vi "zero_FGV.vi"(7 "comandos":enum16{"Set", "Zerar?"}(ring)=enum."Zerar?", 11 "Value":bool) -> (3 "Zerar?":bool)   [LabVIEW 2018]
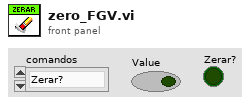
[diagram p1: front panel]
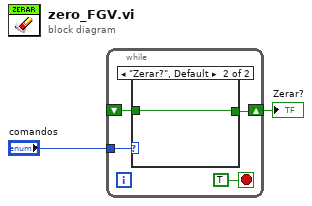
[diagram p0: block diagram]
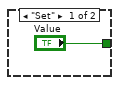
[diagram p2: hidden frame]
diagram:
  n1 = while {
    tunnel: "comandos" -> [w5]
    shift-right: [w4] -> w1
    shift-left: _ -> [w3]
    stop <- TRUE stop-if-true
    n2 = case shown="\"Zerar?\", Default" w5 {
      tunnel: ["Value" w8] -> w4
      tunnel: w3 -> [_ w8]
      frame "Set" {
      }
      frame "Zerar?", Default {
      }
    }
  }
  "Zerar?" <- w1
